vi "Send Shutdown.vi"(8 "error in (no error)":errorcluster, 11 "Dispatcher Interface in":refnum<class "Dispatcher Interface.lvclass">) -> (0 "error out":errorcluster, 3 "Dispatcher Interface out":refnum<class "Dispatcher Interface.lvclass">)   [LabVIEW 2017, in "DSF Core.lvlib" / "Dispatcher Interface.lvclass"]
uses:
  Dispatcher Interface.lvclass
  C:/Git/DSF/Data Sharing Framework Core/Classes/Interfaces/Interface/Interface.lvclass
  Command Data.ctl
  Command.ctl
  Parameters.ctl
  Interface/Interface.lvclass/Interface.ctl
  Response.ctl
  Write Dispatcher Command.vi
  Interface/Send Command.vi
  Interface/Write RT FIFO.vi
  Class Name.vi
  VIs/VI Name.vi
  Command Timeout.vi
  Read Dispatcher Response.vi
  Read Dispatcher Error.vi
  Invalid Response.vi
  Interface/Interface.lvclass
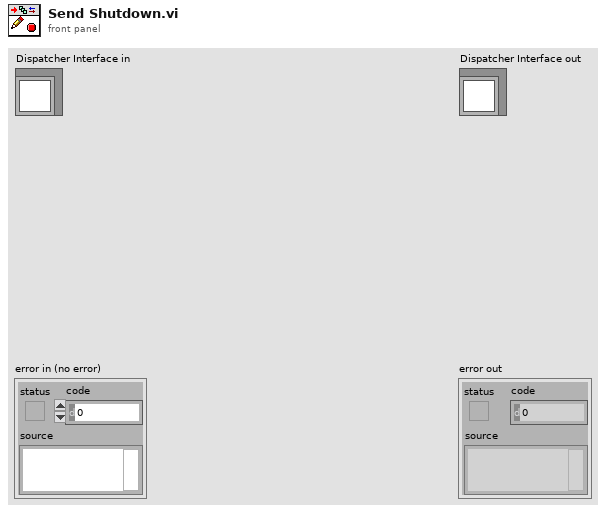
[diagram p1: front panel]
types:
  T1 = typedef "DSF Core.lvlib/Dispatcher Interface.lvclass/Command.ctl" = enum8{"Rx", "Tx", "Set Inline Buffer", "Shutdown"}
  T2 = typedef "DSF Core.lvlib/Dispatcher Interface.lvclass/Command Data.ctl" = cluster{"Command":T1, "Parameters":T3}
  T3 = typedef "DSF Core.lvlib/Dispatcher Interface.lvclass/Parameters.ctl" = cluster{"arg1":u64, "arg2":u64}
  T4 = typedef "DSF Core.lvlib/Dispatcher Interface.lvclass/Response Data.ctl" = cluster{"Response":T5, "Parameters":T3}
  T5 = typedef "DSF Core.lvlib/Dispatcher Interface.lvclass/Response.ctl" = enum8{"General Ack", "Error", "Shutting Down"}
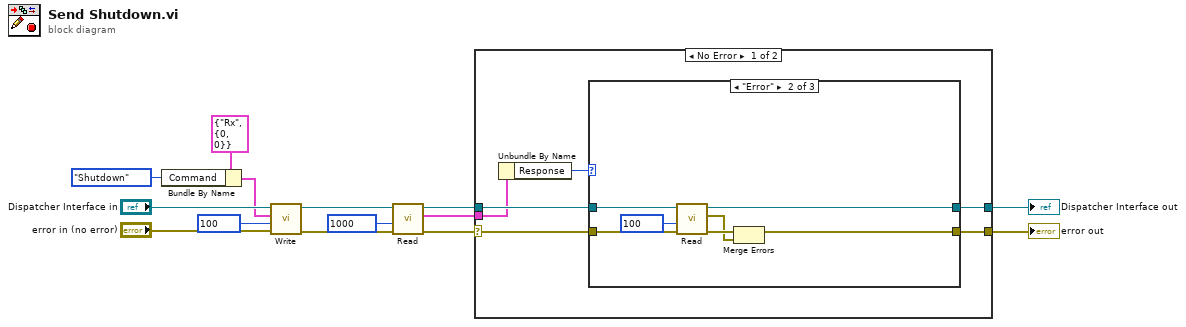
[diagram p0: block diagram]
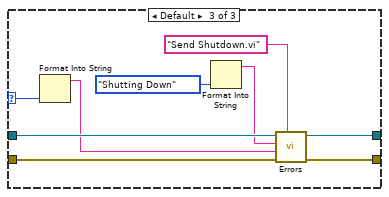
[diagram p3: hidden frame]
diagram:
  n1 = Bundle By Name(cluster=T2 {"Command"=enum."Rx", "Parameters"={"arg1"=0, "arg2"=0}} ("command"), "Command"=Command."Shutdown") -> (w10:T2)
  n2 = call-poly "Write.vi"("error in (no error)"="error in (no error)", "timeout in ms (0)"=100, "command"=w10, "Dispatcher Interface in"="Dispatcher Interface in") -> ("error out"=w6:errorcluster, "Dispatcher Interface out"=w7:refnum<class "Dispatcher Interface.lvclass">)  [unwired: 6 in]
  n3 = call-poly "Read.vi"("error in (no error)"=w6, "timeout in ms (0)"=1000, "Dispatcher Interface in"=w7) -> ("error out"=w4:errorcluster, "response"=w1:T4, "Dispatcher Interface out"=w5:refnum<class "Dispatcher Interface.lvclass">)  [unwired: 5 in, 1 out]
  n4 = case shown="No Error" w4 {
    selector: w4 -> [w15 w39]
    tunnel: [w19 w39] -> w2
    tunnel: w5 -> [w18 w40]
    tunnel: [w17 w40] -> w3
    tunnel: w1 -> [w16 _]
    frame No Error {
      n5 = Unbundle By Name(w16) -> ("Response"=w20:T5)
      n6 = case shown="\"Error\"" w20 {
        selector: w20 -> [_ _ w34]
        tunnel: w15 -> [w21 w28 w37]
        tunnel: [w21 w26 w35] -> w19
        tunnel: w18 -> [w22 w29 w38]
        tunnel: [w22 w25 w36] -> w17
        frame "Shutting Down" {
          # "Valid response."
        }
        frame "Error" {
          n7 = call-poly "Read.vi"("error in (no error)"=w28, "timeout in ms (0)"=100, "Dispatcher Interface in"=w29) -> ("error out"=w24:errorcluster, "error"=w23:errorcluster, "Dispatcher Interface out"=w25:refnum<class "Dispatcher Interface.lvclass">)  [unwired: 6 in]
          n8 = Merge Errors(w24, w23) -> (w26:errorcluster)
        }
        frame Default {
          n9 = Format Into String(w34) -> (resulting string=w33:string)  [unwired: 3 in, 1 out]
          n10 = Format Into String(Response."Shutting Down" ("Response")) -> (resulting string=w32:string)  [unwired: 3 in, 1 out]
          n11 = call-poly "Errors.vi"("error source vi name"="Send Shutdown.vi", "error in (no error)"=w37, "actual response"=w33, "expected response"=w32, "Interface in"=w38) -> ("error out"=w35:errorcluster, "Interface out"=w36:refnum<class "Dispatcher Interface.lvclass">)  [unwired: 5 in]
        }
      }
    }
    frame Error {
      # "Incoming error. Pass through."
    }
  }
  "error out" <- w2
  "Dispatcher Interface out" <- w3
